vi "Unregister Sensor Number.vi"(8 "error in (no error)":errorcluster, 10 "View Enqueuer":refnum<class "Message Enqueuer.lvclass">, 11 "Main Model in":refnum<class "Main Model.lvclass">) -> (0 "error out":errorcluster, 3 "Main Model out":refnum<class "Main Model.lvclass">)   [LabVIEW 2013, in "Main Model.lvlib" / "Main Model.lvclass"]
uses:
  Main Model.lvclass
  <vilib>/ActorFramework/Message Enqueuer/Message Enqueuer.lvclass
  Main Model.lvclass/Main Model.ctl
  <vilib>/ActorFrameworkMVC/View Observer/View Registry/View Registry.lvclass
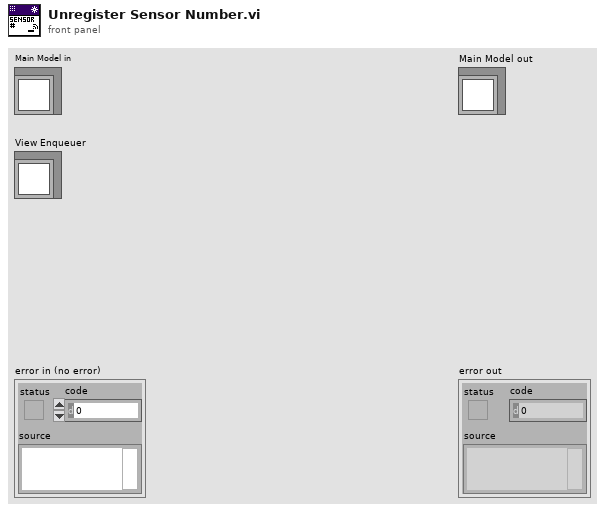
[diagram p1: front panel]
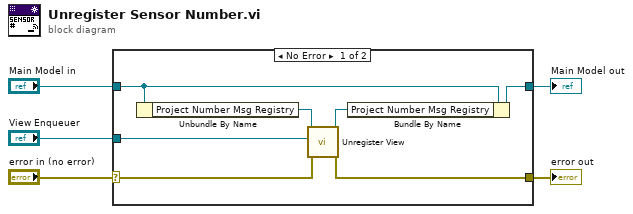
[diagram p0: block diagram]
diagram:
  n1 = case shown="No Error" "error in (no error)" {
    selector: "error in (no error)" -> [w9 w14]
    tunnel: "Main Model in" -> [w12 w13]
    tunnel: "View Enqueuer" -> [w11 _]
    tunnel: [w10 w13] -> w3
    tunnel: [w6 w14] -> w1
    frame No Error {
      n2 = Unbundle By Name(w12) -> ("Project Number Msg Registry"=w8:refnum<class "View Registry.lvclass">)
      n3 = call <vilib>:"Unregister View.vi"("error in (no error)"=w9, "View Enqueuer"=w11, "View Registry in"=w8) -> ("error out"=w6:errorcluster, "View Registry out"=w7:refnum<class "View Registry.lvclass">)  [unwired: 7 in]
      n4 = Bundle By Name(cluster=w12, "Project Number Msg Registry"=w7) -> (w10:refnum<class "Main Model.lvclass">)
    }
    frame Error {
    }
  }
  "error out" <- w1
  "Main Model out" <- w3
